vi "ReadWrite_Function.vi"   [LabVIEW 2016]
uses:
  <vilib>/Platform/TimedLoop/XDataNode/timing_clust.ctl
  <vilib>/Platform/TimedLoop/XDataNode/nitl_modes.ctl
  <vilib>/Platform/TimedLoop/XDataNode/wakeup.ctl
  <vilib>/FPGAPlugInAG/cRIO-9114/niLvFpga_Open_cRIO-9114.vi
  <vilib>/rvi/interface/common/dynamic/niFpgaDynamicAddResources.vi
  <vilib>/FPGAPlugInAG/Dynamic/niLvFpga_Reset_Dynamic.vi
  <vilib>/FPGAPlugInAG/Dynamic/niLvFpga_Run_Dynamic.vi
  <vilib>/Utility/error.llb/Error Cluster From Error Code.vi
  <vilib>/rvi/errors/niLvFpgaAdjustHostInterfaceError.vi
  <vilib>/FPGAPlugInAG/Dynamic/niLvFpga_Close_Dynamic.vi
  <vilib>/rvi/interface/nirviOpenFPGA/nirviOpenFPGA.xnode
  FPGA Bitfiles/Test_FPGATarget_CANBasic(FPGA)_-t83YMbv2CI.lvbitx
  CAN Basic (FPGA).vi
  <vilib>/rvi/interface/nirviMethod/nirviMethod.xnode
  <vilib>/platform/TimedLoop/XDataNode/XDataNode.xnode
  <vilib>/rvi/interface/nirviReadWriteControl/nirviReadWriteControl.xnode
  <vilib>/rvi/interface/nirviCloseFPGA/nirviCloseFPGA.xnode
  <vilib>/Platform/TimedLoop/XDataNode/XDNodeRunTimeDep.lvlib
  NiFpgaLv.dll
  <vilib>/rvi/interface/Simulation/niFpgaSimulationCallBeginRW.vi
types:
  T1 = cluster{"timestamp high":u32, "timestamp low":u32, "identifier":u32, "type":enum8{"Data Frame", "Remote Frame", "(reserved)", "(reserved) ", "(reserved)  ", "(reserved)   ", "Bus Error", "Transceiver Fault"}, "info A":u8, "info B":u8, "data length":u8, "data":u8[]}
  T2 = typedef "XDNodeRunTimeDep.lvlib/timing_clust.ctl" = cluster{"Expected End [f-1]":u64, "Actual End [f-1]":u64, "Finished Late? [f-1]":bool, "Expected End [i-1]":u64, "Actual End [i-1]":u64, "Finished Late? [i-1]":bool, "Expected Start [i]":u64, "Actual Start [i]":u64, "Expected Start [f]":u64, "Actual Start [f]":u64, "Source Name":string, "Structure Name":string, "Period":i64, "Deadline":i64, "Offset":i64, "Start":i64, "Priority":i32, "Timeout":i32, "Mode":T3, "Wakeup Reason":T4, "Error":errorcluster, "Source Type":string, "Secondary Source Type":string, "Global End Time":u64, "Global Start Time":u64, "Frame Duration":u64, "Iteration Duration":u64, "Assigned CPU":i32, "I/O Scan Engine Mode":u32}
  T3 = typedef "XDNodeRunTimeDep.lvlib/nitl_modes.ctl" = enum32{"No Change", "Process missed periods, maintain original phase", "Discard missed periods, maintain original phase", "Process missed periods, ignore original phase", "Discard missed periods, ignore original phase"}
  T4 = typedef "XDNodeRunTimeDep.lvlib/wakeup.ctl" = enum32{"Normal", "Aborted", "Asynchronous wakeup", "Timing source error", "Timed loop error", "Timeout"}
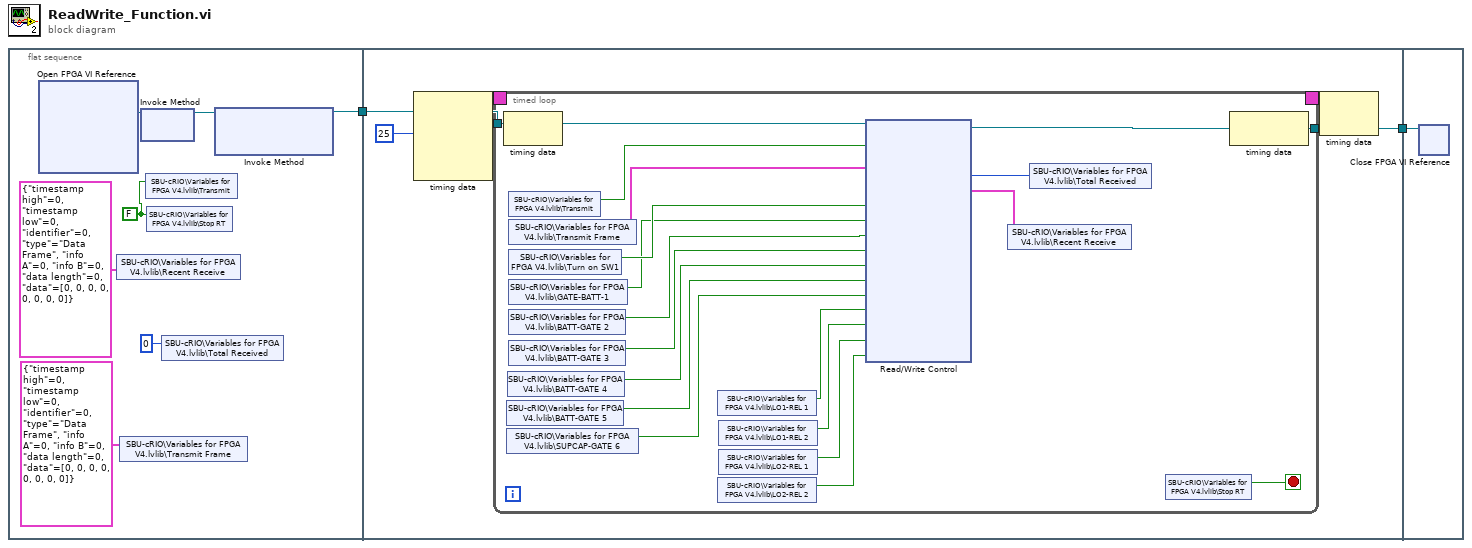
[diagram p0: block diagram]
diagram:
  n1 = flat-sequence {
    tunnel: [w8] -> w2
    tunnel: w2 -> [w14]
    tunnel: [w10] -> w1
    tunnel: w1 -> [w39]
    frame #0 {
      w7 = FALSE ("Stop RT")
      n2 = xnode "Open FPGA VI Reference"() -> ("FPGA VI Reference Out"=w3:refnum<k20>)  [unwired: 2 in, 1 out]
      n3 = shared-variable "SBU-cRIO\\Variables for FPGA V4.lvlib\\Recent Receive"(T1 {"timestamp high"=0, "timestamp low"=0, "identifier"=0, "type"=enum."Data Frame", "info A"=0, "info B"=0, "data length"=0, "data"=[0, 0, 0, 0, 0, 0, 0, 0]} ("Recent Receive")) -> ()  [unwired: 1 in, 1 out]
      n4 = shared-variable "SBU-cRIO\\Variables for FPGA V4.lvlib\\Transmit Frame"(T1 {"timestamp high"=0, "timestamp low"=0, "identifier"=0, "type"=enum."Data Frame", "info A"=0, "info B"=0, "data length"=0, "data"=[0, 0, 0, 0, 0, 0, 0, 0]} ("Transmit Frame")) -> ()  [unwired: 1 in, 1 out]
      n5 = xnode "Invoke Method"("FPGA VI Reference In"=w3) -> ("FPGA VI Reference Out"=w9:refnum<k20>)  [unwired: 1 in, 1 out]
      n6 = shared-variable "SBU-cRIO\\Variables for FPGA V4.lvlib\\Transmit"(w7) -> ()  [unwired: 1 in, 1 out]
      n7 = shared-variable "SBU-cRIO\\Variables for FPGA V4.lvlib\\Stop RT"(w7) -> ()  [unwired: 1 in, 1 out]
      n8 = shared-variable "SBU-cRIO\\Variables for FPGA V4.lvlib\\Total Received"(u32 0 ("Total Received")) -> ()  [unwired: 1 in, 1 out]
      n9 = xnode "Invoke Method"("FPGA VI Reference In"=w9) -> ("FPGA VI Reference Out"=w8:refnum<k20>)  [unwired: 2 in, 1 out]
    }
    frame #1 {
      n10 = node-c288(i64 25 ("Period")) -> (w13:T2)  [unwired: 3 in]
      n11 = timed-loop {
        tunnel: w14 -> [w32]
        tunnel: [w30] -> w10
        timing: w13 -> [_]
        timing-out: [_] -> w12
        stop <- w31 stop-if-true
        n12 = node-c288() -> ()  [unwired: 1 in, 1 out]
        n13 = shared-variable "SBU-cRIO\\Variables for FPGA V4.lvlib\\BATT-GATE 5"() -> (w22:bool)  [unwired: 1 in, 1 out]
        n14 = shared-variable "SBU-cRIO\\Variables for FPGA V4.lvlib\\SUPCAP-GATE 6"() -> (w21:bool)  [unwired: 1 in, 1 out]
        n15 = shared-variable "SBU-cRIO\\Variables for FPGA V4.lvlib\\BATT-GATE 4"() -> (w23:bool)  [unwired: 1 in, 1 out]
        n16 = shared-variable "SBU-cRIO\\Variables for FPGA V4.lvlib\\Transmit"() -> (w29:bool)  [unwired: 1 in, 1 out]
        n17 = shared-variable "SBU-cRIO\\Variables for FPGA V4.lvlib\\Transmit Frame"() -> (w28:T1)  [unwired: 1 in, 1 out]
        n18 = shared-variable "SBU-cRIO\\Variables for FPGA V4.lvlib\\Turn on SW1"() -> (w25:bool)  [unwired: 1 in, 1 out]
        n19 = shared-variable "SBU-cRIO\\Variables for FPGA V4.lvlib\\GATE-BATT-1"() -> (w15:bool)  [unwired: 1 in, 1 out]
        n20 = shared-variable "SBU-cRIO\\Variables for FPGA V4.lvlib\\BATT-GATE 2"() -> (w16:bool)  [unwired: 1 in, 1 out]
        n21 = shared-variable "SBU-cRIO\\Variables for FPGA V4.lvlib\\BATT-GATE 3"() -> (w24:bool)  [unwired: 1 in, 1 out]
        n22 = shared-variable "SBU-cRIO\\Variables for FPGA V4.lvlib\\LO1-REL 1"() -> (w20:bool)  [unwired: 1 in, 1 out]
        n23 = shared-variable "SBU-cRIO\\Variables for FPGA V4.lvlib\\LO2-REL 2"() -> (w17:bool)  [unwired: 1 in, 1 out]
        n24 = shared-variable "SBU-cRIO\\Variables for FPGA V4.lvlib\\LO1-REL 2"() -> (w19:bool)  [unwired: 1 in, 1 out]
        n25 = shared-variable "SBU-cRIO\\Variables for FPGA V4.lvlib\\LO2-REL 1"() -> (w18:bool)  [unwired: 1 in, 1 out]
        n26 = xnode "Read/Write Control"("FPGA VI Reference In"=w32, "Transmit"=w29, "Transmit Frame"=w28, "Gatedriver1"=w25, "GATE-BATT-1"=w15, "BATT-GATE 2"=w16, "BATT-GATE 3"=w24, "BATT-GATE 4"=w23, "BATT-GATE 5"=w22, "SUPCAP-GATE 6"=w21, "LO1-REL 1"=w20, "LO1-REL 2"=w19, "LO2-REL 1"=w18, "LO2-REL 2"=w17) -> ("FPGA VI Reference Out"=w30:refnum<k20>, "Total Received"=w27:u32, "Recent Receive"=w26:T1)  [unwired: 1 in, 1 out]
        n27 = shared-variable "SBU-cRIO\\Variables for FPGA V4.lvlib\\Recent Receive"(w26) -> ()  [unwired: 1 in, 1 out]
        n28 = shared-variable "SBU-cRIO\\Variables for FPGA V4.lvlib\\Total Received"(w27) -> ()  [unwired: 1 in, 1 out]
        n29 = shared-variable "SBU-cRIO\\Variables for FPGA V4.lvlib\\Stop RT"() -> (w31:bool)  [unwired: 1 in, 1 out]
        n30 = node-c288() -> ()  [unwired: 1 in, 1 out]
      }
      n31 = node-c288(w12) -> ()  [unwired: 1 out]
    }
    frame #2 {
      n32 = xnode "Close FPGA VI Reference"("FPGA VI Reference In"=w39) -> ()  [unwired: 1 in, 1 out]
    }
  }
